vi "Shift Point by Time.vi"(5 "Buffer Length":i32, 7 "dt":dbl, 8 "error in (no error)":errorcluster, 10 "Time":dbl, 11 "Data Point in":T1) -> (0 "error out":errorcluster, 2 "Samples shifted":i32, 3 "Data Point out":T1)   [LabVIEW 2015, in "Waveform Buffer.lvclass"]
uses:
  Waveform Buffer.lvclass
  Data Point.ctl
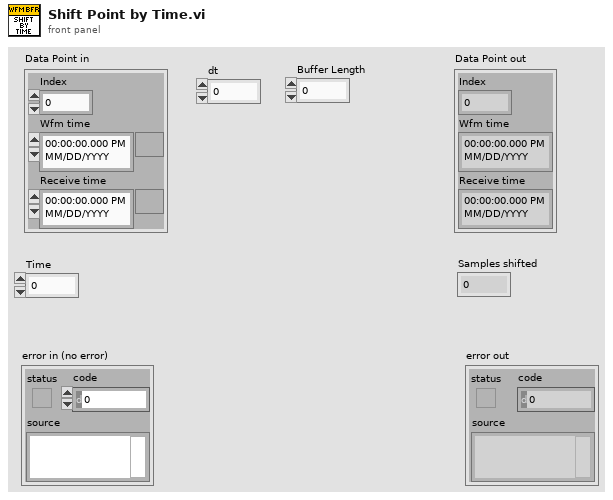
[diagram p1: front panel]
types:
  T1 = typedef "Waveform Buffer.lvclass/Data Point.ctl" = cluster{"Index":i32, "Wfm time":timestamp, "Receive time":timestamp}
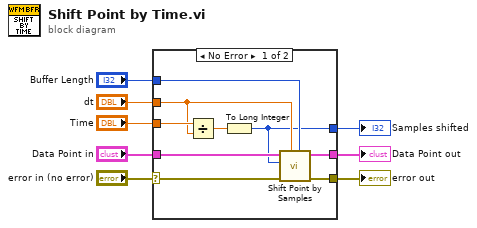
[diagram p0: block diagram]
diagram:
  n1 = case shown="No Error" "error in (no error)" {
    selector: "error in (no error)" -> [w15 w19]
    tunnel: [w14 w19] -> w7
    tunnel: [w13 w18] -> w5
    tunnel: "Data Point in" -> [w12 w18]
    tunnel: "Time" -> [w17 _]
    tunnel: "dt" -> [w11 _]
    tunnel: [w9 _] -> w2
    tunnel: "Buffer Length" -> [w10 _]
    frame No Error {
      n2 = Divide(x=w17, y=w11) -> (x/y=w16:dbl)
      n3 = To Long Integer(number=w16) -> (32bit integer=w9:i32)
      n4 = call "Shift Point by Samples.vi"("Buffer Length"=w10, "dt"=w11, "error in (no error)"=w15, "Samples"=w9, "Data Point in"=w12) -> ("error out"=w14:errorcluster, "Data Point out"=w13:T1)  [unwired: 4 in, 1 out]
    }
    frame Error {
    }
  }
  "error out" <- w7
  "Samples shifted" <- w2
  "Data Point out" <- w5
